vi "Merge Color With Image Data.vi"(8 "error in (no error)":errorcluster, 10 "Color":u32(colorbox)=16777215, 11 "Image Data in":T1) -> (0 "error out":errorcluster, 3 "Image Data out":T1)   [LabVIEW 2011]
doc: "This VI will take <B>Image Data in</B> and create <B>Image Data out</B> which is the same image with a 50% merge with <b>Color</b> from the original. This will make the image appear greyed out or disabled. If the image data is not 32Bit it will be converted to it with the assumption that all pixels are solid and not transparent.\n\n-------------\nDeveloped by Brian Hoover (hooovahh)"
uses:
  <vilib>/picture/picture.llb/imagedata.ctl
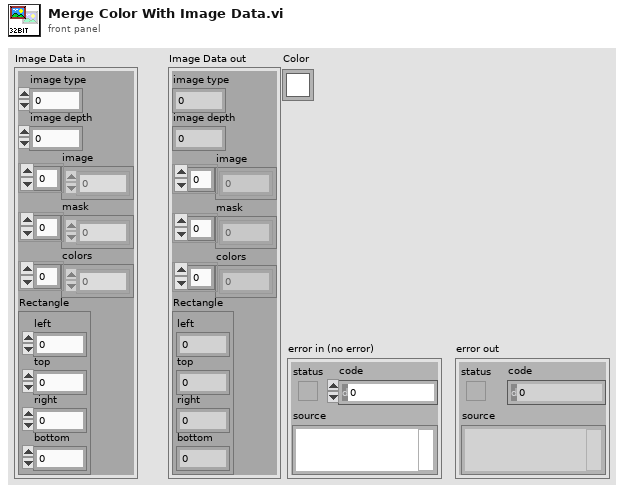
[diagram p1: front panel]
types:
  T1 = typedef "imagedata.ctl" = cluster{"image type":i32, "image depth":i32, "image":u8[], "mask":u8[], "colors":u32[], "Rectangle":cluster{"left":i16, "top":i16, "right":i16, "bottom":i16}}
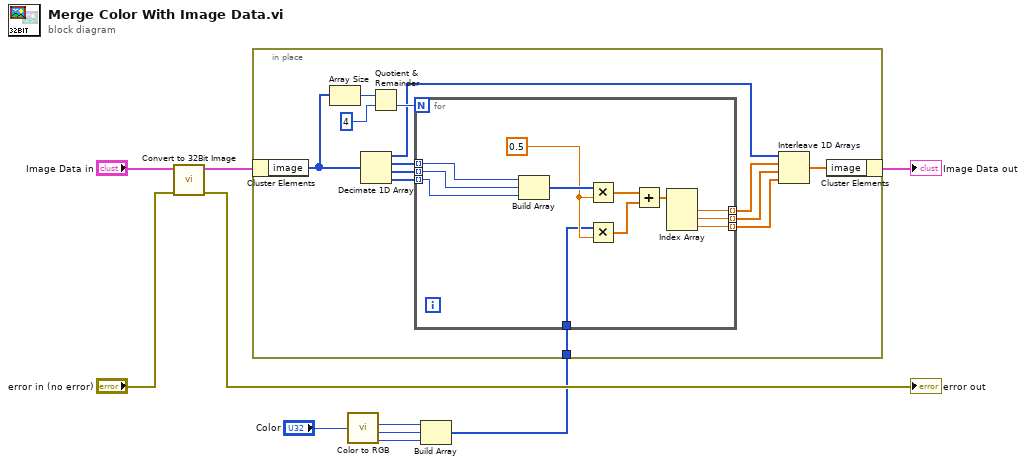
[diagram p0: block diagram]
diagram:
  n1 = call "Convert to 32Bit Image.vi"("error in (no error)"="error in (no error)", "Image Data"="Image Data in") -> ("error out"=→"error out":errorcluster, "32Bit Image Data Out"=w8:T1)  [unwired: 8 in]
  n2 = call <vilib>:"Color to RGB.vi"("Color"="Color") -> ("R"=w5:u8, "G"=w4:u8, "B"=w3:u8)  [unwired: 1 out]
  n3 = Build Array(w5, w4, w3) -> (w2:u8[])
  n4 = in-place {
    in-place-border: w2 -> [w15]
    n5 = in-place-cluster #1(w8) -> ("image"=w20:u8[])
    n6 = Array Size(array=w20) -> (size(s)=w22:i32)
    n7 = Decimate 1D Array(w20) -> (w11:u8[], w19:u8[], w18:u8[], w17:u8[])
    n8 = Quotient & Remainder(x=w22, y=4) -> (floor(x/y)=w21:i32)  [unwired: 1 out]
    n9 = for {
      N: w21 -> [_]
      tunnel: w19 -> [w30] mode=indexing
      tunnel: w18 -> [w29] mode=indexing
      tunnel: w17 -> [w28] mode=indexing
      tunnel: w15 -> [w27]
      tunnel: [w26] -> w14 mode=indexing
      tunnel: [w25] -> w13 mode=indexing
      tunnel: [w24] -> w12 mode=indexing
      w31 = 0.5 ("Slide 2")
      n10 = Build Array(w30, w29, w28) -> (w33:u8[])
      n11 = Multiply(x=w33, y=w31) -> (x*y=w32:dbl[])
      n12 = Multiply(x=w27, y=w31) -> (x*y=w34:dbl[])
      n13 = Add(x=w32, y=w34) -> (x+y=w35:dbl[])
      n14 = Index Array(array=w35) -> (element #1=w26:dbl, element #2=w25:dbl, element #3=w24:dbl)  [unwired: 3 in]
    }
    n15 = Interleave 1D Arrays(w11, w14, w13, w12) -> (w16:dbl[])
    n16 = in-place-cluster #1("image"=w16) -> (→"Image Data out":T1)
  }
